vi "Runtime Test.vi"() -> ()   [LabVIEW 2015, in "Increment tests.lvlib"]
doc: "This VI shows an example for how to test the Runtime functionality of the module. This will need to be modified according to module functionality."
uses:
  Increment tests.lvlib
  module/execution/Increment runtime.lvclass
  <vilib>/NI/Tag Bus/dictionary/data dictionary.lvclass/data dictionary.ctl
  <vilib>/NI/Tag Bus/dictionary/lookup polymorphs/locate double.vi
  <vilib>/NI/Tag Bus/table/data polymorphs/write one/write Double.vi
  <vilib>/NI/Tag Bus/table/data polymorphs/read one/read Double.vi
  <vilib>/NI/Tag Bus/dictionary/search/find data index.vi
  <vilib>/NI/Tag Bus/dictionary/search/search string list.vi
  <vilib>/NI/Tag Bus/dictionary/tag not found.vi
  module/configuration/Increment configuration.lvclass
  <vilib>/NI/Tag Bus/dictionary/data dictionary.lvclass
  <vilib>/NI/Tag Bus/table/data table.lvlib
panel:
  out "Names":string[](array[string])
  out "Processing Result":dbl
  in  "Processing Parameters":dbl
  out "error":errorcluster
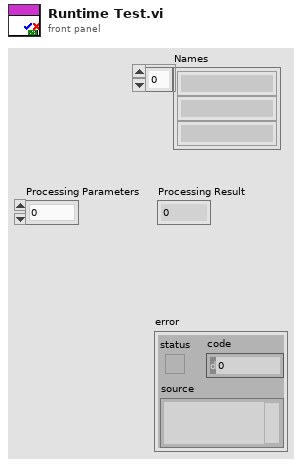
[diagram p1: front panel]
types:
  T1 = typedef "TBM channel.lvclass/data tables.ctl" = cluster{"input data":T2, "processing parameter":T2, "processing result":T2, "output data":T2}
  T2 = typedef "tag bus.lvlib/dictionary table pair.ctl" = cluster{"data dictionary":refnum<class "data dictionary.lvclass">, "data table":T3}
  T3 = typedef "tag bus.lvlib/data table.lvlib/data table.ctl" = cluster{"Double":dbl[], "Single":sgl[], "I64":i64[], "I32":i32[], "I16":i16[], "I8":i8[], "U64":u64[], "U32":u32[], "U16":u16[], "U8":u8[], "Boolean":bool[], "String":string[], "Array of Double":cluster{"DBL Array":dbl[]}[], "Array of Single":cluster{"SGL Array":sgl[]}[], "Array of I64":cluster{"I64 Array":i64[]}[], "Array of I32":cluster{"I32 Array":i32[]}[], "Array of I16":cluster{"I16 Array":i16[]}[], "Array of I8":cluster{"I8 Array":i8[]}[], "Array of U64":cluster{"U64 Array":u64[]}[], "Array of U32":cluster{"U32 Array":u32[]}[], "Array of U16":cluster{"U16 Array":u16[]}[], "Array of U8":cluster{"U8 Array":u8[]}[], "Array of Boolean":cluster{"Boolean Array":bool[]}[], "Array of String":cluster{"String Array":string[]}[]}
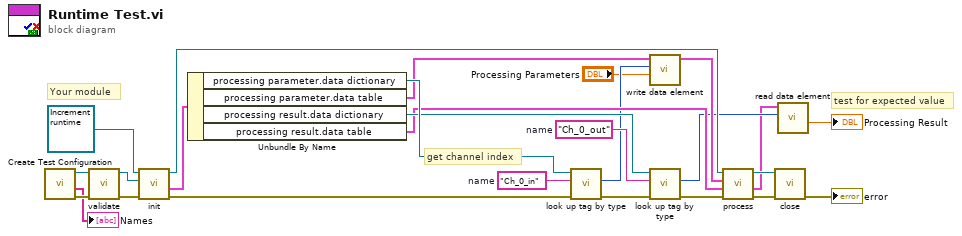
[diagram p0: block diagram]
diagram:
  w7 = "Ch_0_in"  # name
  w9 = "Ch_0_out"  # name
  # "test for expected value"
  # "get channel index"
  # "Your module"
  n1 = call "Create Test Configuration.vi"() -> ("error out"=w22:errorcluster, "Names"=→"Names":string[], "Module Configuration"=w23:refnum<class "Increment configuration.lvclass">)  [unwired: 6 in, 3 out]
  n2 = call-dynamic "validate.vi"("error in"=w22, "Increment configuration in"=w23) -> ("error out"=w25:errorcluster, "Increment configuration out"=w24:refnum<class "Increment configuration.lvclass">)  [unwired: 8 in]
  n3 = call-dynamic "init.vi"("error in"=w25, "TBM module configuration in"=w24, "Increment runtime in"=refnum<class "Increment runtime.lvclass"> refnum ("tag bus configurable plugin module")) -> ("error out"=w14:errorcluster, "data allocations"=w15:T1, "Increment runtime out"=w16:refnum<class "Increment runtime.lvclass">)  [unwired: 5 in, 1 out]
  n4 = Unbundle By Name(w15) -> ("processing parameter.data dictionary"=w21:refnum<class "data dictionary.lvclass">, "processing parameter.data table"=w20:T3, "processing result.data dictionary"=w18:refnum<class "data dictionary.lvclass">, "processing result.data table"=w17:T3)
  n5 = call-poly <vilib>:"look up tag by type.vi"("error in"=w14, "name"=w7, "data dictionary in"=w21) -> ("error out"=w5:errorcluster, "index"=w8:i32)  [unwired: 6 in, 1 out]
  n6 = call-poly <vilib>:"write data element.vi"("value"="Processing Parameters", "index"=w8, "data table in"=w20) -> ("data table out"=w11:T3)  [unwired: 8 in]
  n7 = call-poly <vilib>:"look up tag by type.vi"("error in"=w5, "name"=w9, "data dictionary in"=w18) -> ("error out"=w4:errorcluster, "index"=w10:i32)  [unwired: 6 in, 1 out]
  n8 = call-dynamic "process.vi"("error in"=w4, "result allocation"=w17, "parameters"=w11, "module in"=w16) -> ("error out"=w12:errorcluster, "results"=w6:T3, "module out"=w13:refnum<class "Increment runtime.lvclass">)  [unwired: 4 in, 1 out]
  n9 = call-dynamic "close.vi"("error in"=w12, "Increment runtime in"=w13) -> ("error out"=→"error":errorcluster)  [unwired: 9 in]
  n10 = call-poly <vilib>:"read data element.vi"("index"=w10, "data table in"=w6) -> ("value"=→"Processing Result":dbl)  [unwired: 8 in, 1 out]
